vi "Parallel centroid calc (Optimized Performance) ajg.vi"() -> ()   [LabVIEW 2020]
doc: "The Parallel Processing (Optimized Performance) example shows how to process multiple images in parallel when using a ring acquisition. Images acquired from a camera are stored in a ring buffer and references to each image are pushed to a queue. Each worker loop removes a reference from the queue and processes the image.\n\nIn this example, image processing is simulated by a time delay that can be adjusted while the VI is running. When processing is complete, <B>IMAQdx Release Image</B> must be called in order to free space in the ring buffer."
uses:
  <vilib>/vision/driver/IMAQdx.llb/IMAQdx Acquisition Mode.ctl
  <vilib>/vision/Image Controls.llb/IMAQ Image.ctl
  <vilib>/vision/driver/IMAQdx.llb/IMAQdx Buffer Number Mode.ctl
  <vilib>/vision/driver/NI_Vision_Acquisition_Software.lvlib
  <resource>/objmgr/imaqdx.rc
panel:
  out "Images Saved Per Second":dbl
  out "Images Acquired Per Second":dbl
  out "Images Behind":u32
  in  "save path":path
  in  "Range":cluster{"Lower value":sgl, "Upper value":sgl}={"Lower value"=128.0, "Upper value"=255.0} {"Upper value" format="%.2f"; "Lower value" format="%.2f"}
  out "Lost Buffer Count":u32
  in  "Processing Delay (s)":dbl(slide)=0.1 scale=0.0..1.0
  out "Images Processed":u32
  out "Current Buffer Number":u32
  in  "Processing Delay (s)":dbl(slide)=0.2 scale=0.0..1.0
  out "Images Processed":u32
  out "Current Buffer Number":u32
  in  "Number of Images":i32=30
  out "Images in Queue":i32
  out "Images Processed":u32
  out "Current Buffer Number":u32
  in  "Camera Name":refnum<k21> caption="IMAQdx Session"
  in  "Stop":bool
  # "Overview: Demonstrates how to process multiple extracted images in parallel when using a ring acquisition.\nRequirements: Vision Acquisition Software\nInstructions:\n1. Select the Camera Name\n2. Run the VI"
  # "Worker Loop 1"
  # "Worker Loop 3"
  # "Worker Loop 2"
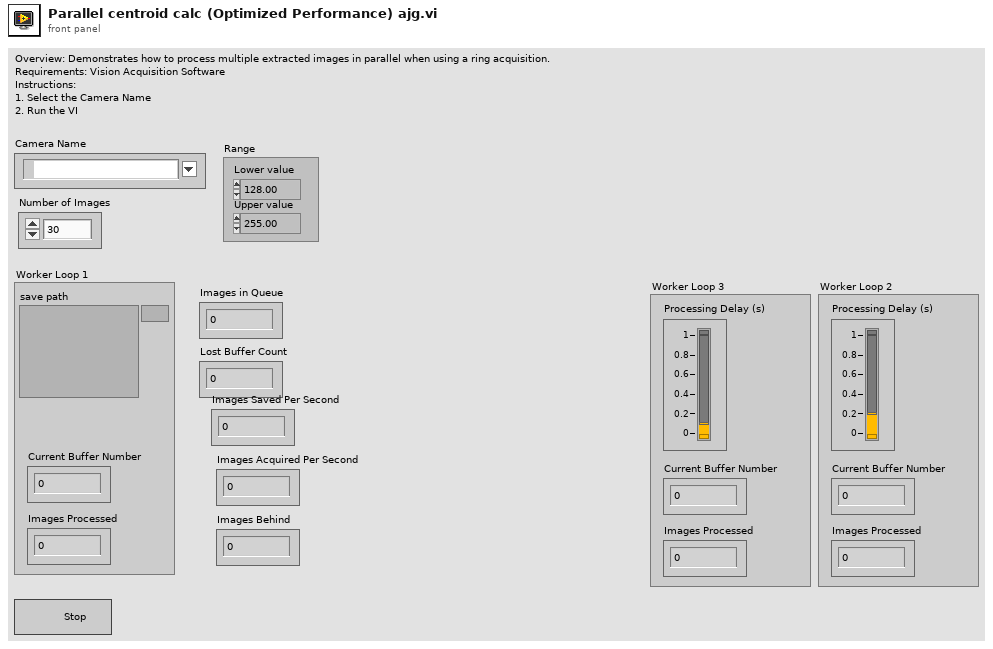
[diagram p1: front panel]
types:
  T1 = enum16{"open", "open or create", "create or replace", "create", "open (read-only)"}
  T2 = typedef "IMAQ Image.ctl" = refnum<image>
  T3 = typedef "NI_Vision_Acquisition_Software.lvlib/IMAQdx Acquisition Mode.ctl" = enum32{"One Shot", "Continuous"}
  T4 = typedef "IMAQdx.ctl" = refnum<k21>
  T5 = typedef "NI_Vision_Acquisition_Software.lvlib/IMAQdx Buffer Number Mode.ctl" = enum32{"Next", "Last", "Buffer Number", "Every", "Last New"}
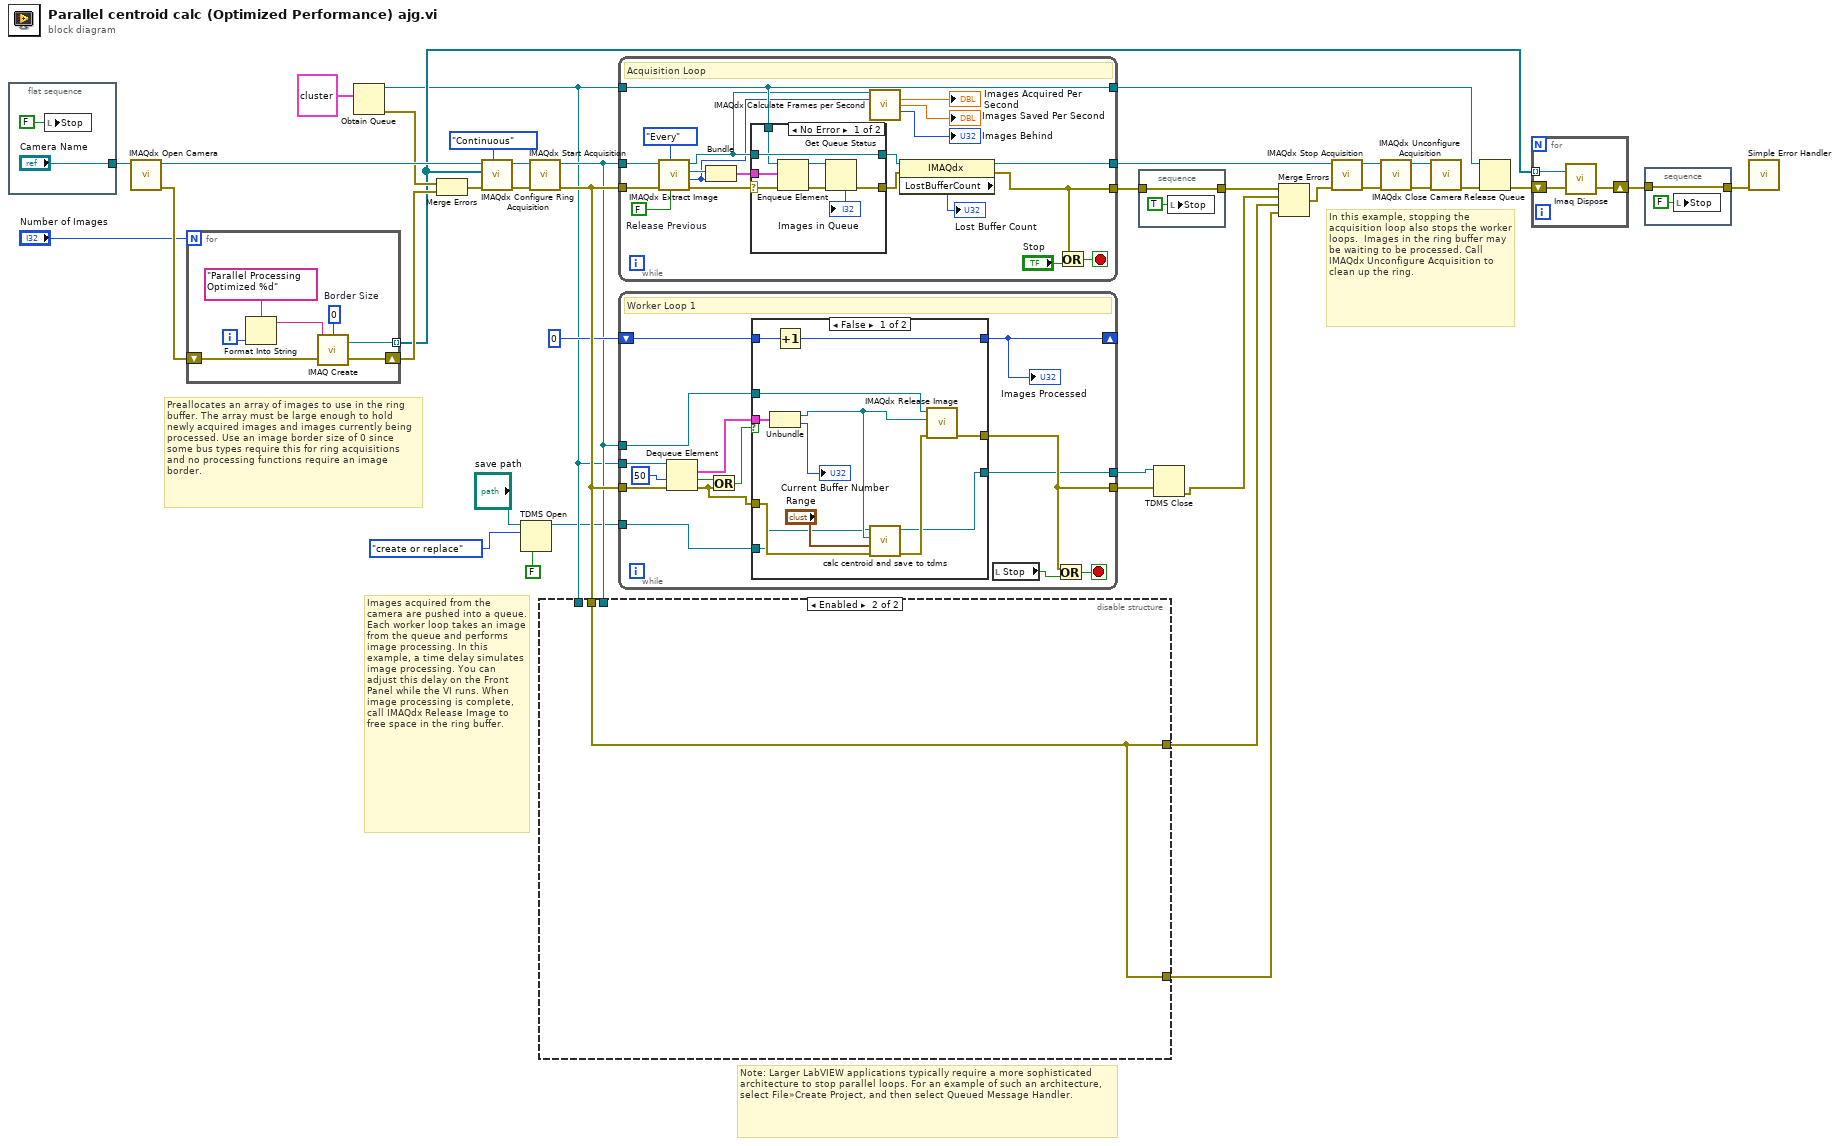
[diagram p0: block diagram]
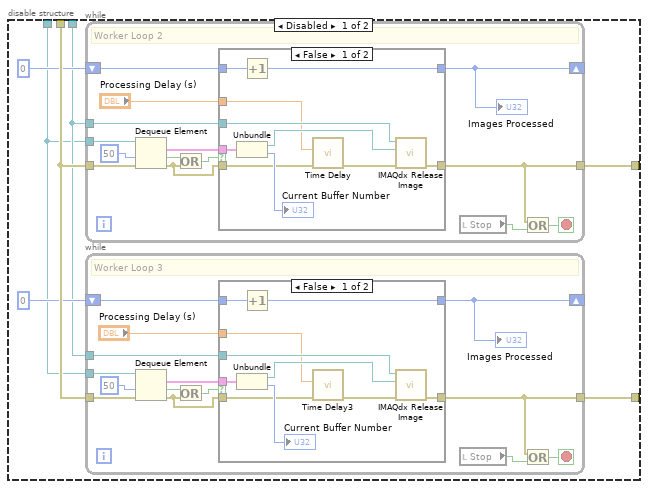
[diagram p2: hidden frame]
diagram:
  # "In this example, stopping the acquisition loop also stops the worker loops.  Images in the ring buffer may be waiting to be processed. Call IMAQdx Unconfigure Acquisition to clean up the ring."
  # "Images acquired from the camera are pushed into a queue. Each worker loop takes an image from the queue and performs image processing. In this example, a time delay simulates image processing. You can adjust this delay on the Front Panel while the VI runs. When image processing is complete, call IMAQdx Release Image to free space in the ring buffer."
  # "Preallocates an array of images to use in the ring buffer. The array must be large enough to hold newly acquired images and images currently being processed. Use an image border size of 0 since some bus types require this for ring acquisitions and no processing functions require an image border."
  # "Note: Larger LabVIEW applications typically require a more sophisticated architecture to stop parallel loops. For an example of such an architecture, select File»Create Project, and then select Queued Message Handler."
  n1 = flat-sequence {
    tunnel: ["Camera Name"] -> w36
    frame #0 {
      n2 = local write "Stop"(FALSE ("Stop")) -> ()
    }
  }
  n3 = call <vilib>:"IMAQdx Open Camera.vi"("Session In"=w36) -> ("error out"=w29:errorcluster, "Session Out"=w28:T4)  [unwired: 2 in, 7 out]
  n4 = for {
    N: "Number of Images" -> [_]
    tunnel: [w46] -> w19 mode=indexing
    shift-right: [w45] -> w24
    shift-left: w29 -> [w47]
    i -> [w44]
    w41 = 0  # Border Size
    n5 = Format Into String(format string="Parallel Processing Optimized %d" ("Image Name"), w44) -> (resulting string=w43:string)  [unwired: 2 in, 1 out]
    n6 = call "IMAQ Create"("Border Size"=w41, "Image Name"=w43, "error in (no error)"=w47) -> ("New Image"=w46:T2, "error out"=w45:errorcluster)  [unwired: 1 in, 1 out]
  }
  n7 = Obtain Queue(element data type=cluster{"Image Out":T2, "Buffer Number Out":u32} {"Image Out"=refnum, "Buffer Number Out"=0}) -> (queue out=w12:refnum<queue>, error out=w23:errorcluster)  [unwired: 4 in, 1 out]
  n8 = Merge Errors(w23, w24) -> (w25:errorcluster)
  n9 = call <vilib>:"IMAQdx Configure Ring Acquisition.vi"("Mode"=IMAQdx_Acquisition_Mode."Continuous" ("Continuous?"), "error in"=w25, "Images"=w19, "Session In"=w28) -> ("error out"=w30:errorcluster, "Session Out"=w31:T4)  [unwired: 5 in, 1 out]
  n10 = TDMS Open(6:FALSE ("disable buffering (T)"), 10:T1."create or replace" ("operation"), 11:"save path") -> (3:w4:refnum<k34>)  [unwired: 4 in, 1 out]
  n11 = call <vilib>:"IMAQdx Start Acquisition.vi"("error in"=w30, "Session In"=w31) -> ("error out"=w38:errorcluster, "Session Out"=w15:T4)  [unwired: 8 out]
  n12 = disable-structure shown="Enabled" {
    disable-tunnel: w38 -> [w54 w107]
    disable-tunnel: w15 -> [w51 _]
    disable-tunnel: [w50 w107] -> w14
    disable-tunnel: [w49 w107] -> w13
    disable-tunnel: w12 -> [w48 _]
    frame Disabled {
      n13 = while {
        tunnel: [w87] -> w50
        tunnel: w48 -> [w91]
        tunnel: w51 -> [w90]
        shift-right: [w85] -> _
        shift-left: u32 0 -> [w89]
        tunnel: w54 -> [w84]
        stop <- w93 stop-if-true
        # "Worker Loop 2"
        n14 = Dequeue Element(queue=w91, timeout in ms (-1)=50 ("timeout in ms"), error in (no error)=w84) -> (element=w92:cluster{"Image Out":T2, "Buffer Number Out":u32}, timed out?=w81:bool, error out=w82:errorcluster)  [unwired: 1 out]
        n15 = Or(x=w81, y=w82) -> (x .or. y?=w83:bool)
        n16 = case shown="False" w83 {
          tunnel: w92 -> [w104 _]
          tunnel: [w103 w105] -> w87
          tunnel: "Processing Delay (s)" -> [w97 _]
          tunnel: w90 -> [w100 _]
          tunnel: w89 -> [w99 w106]
          tunnel: [w98 w106] -> w85
          tunnel: w82 -> [w95 w105]
          frame False {
            n17 = Unbundle(w104) -> ("Image Out"=w101:T2, "Buffer Number Out"=→"Current Buffer Number":u32)
            n18 = Increment(x=w99) -> (x+1=w98:u32)
            n19 = call "Time Delay"("error in (no error)"=w95, "Delay Time (s)"=w97) -> ("error out"=w102:errorcluster)  [unwired: 9 in]
            n20 = call <vilib>:"IMAQdx Release Image.vi"("error in"=w102, "Image"=w101, "Session In"=w100) -> ("error out"=w103:errorcluster)  [unwired: 7 in, 1 out]
          }
          frame True {
            # "Empty queue or error.\nNothing to process."
          }
        }
        "Images Processed" <- w85
        n21 = local read "Stop"() -> (w88:bool)
        n22 = Or(x=w87, y=w88) -> (x .or. y?=w93:bool)
      }
      n23 = while {
        tunnel: [w61] -> w49
        tunnel: w48 -> [w65]
        tunnel: w51 -> [w64]
        shift-right: [w59] -> _
        shift-left: u32 0 -> [w63]
        tunnel: w54 -> [w58]
        stop <- w67 stop-if-true
        # "Worker Loop 3"
        n24 = Dequeue Element(queue=w65, timeout in ms (-1)=50 ("timeout in ms"), error in (no error)=w58) -> (element=w66:cluster{"Image Out":T2, "Buffer Number Out":u32}, timed out?=w57:bool, error out=w55:errorcluster)  [unwired: 1 out]
        n25 = Or(x=w57, y=w55) -> (x .or. y?=w56:bool)
        n26 = case shown="False" w56 {
          tunnel: w66 -> [w78 _]
          tunnel: [w77 w79] -> w61
          tunnel: "Processing Delay (s)" -> [w71 _]
          tunnel: w64 -> [w74 _]
          tunnel: w63 -> [w73 w80]
          tunnel: [w72 w80] -> w59
          tunnel: w55 -> [w69 w79]
          frame False {
            n27 = Unbundle(w78) -> ("Image Out"=w75:T2, "Buffer Number Out"=→"Current Buffer Number":u32)
            n28 = Increment(x=w73) -> (x+1=w72:u32)
            n29 = call "Time Delay3"("error in (no error)"=w69, "Delay Time (s)"=w71) -> ("error out"=w76:errorcluster)  [unwired: 9 in]
            n30 = call <vilib>:"IMAQdx Release Image.vi"("error in"=w76, "Image"=w75, "Session In"=w74) -> ("error out"=w77:errorcluster)  [unwired: 7 in, 1 out]
          }
          frame True {
            # "Empty queue or error.\nNothing to process."
          }
        }
        "Images Processed" <- w59
        n31 = local read "Stop"() -> (w62:bool)
        n32 = Or(x=w61, y=w62) -> (x .or. y?=w67:bool)
      }
    }
    frame Enabled {
    }
  }
  n33 = while {
    tunnel: w38 -> [w127]
    tunnel: w15 -> [w123]
    tunnel: w12 -> [w114]
    tunnel: [w122] -> w18
    tunnel: [w120] -> w11
    tunnel: [w114] -> w20
    stop <- w119 stop-if-true
    w124 = FALSE  # Release Previous
    # "Acquisition Loop"
    n34 = call <vilib>:"IMAQdx Extract Image.vi"("Release Previous (true)"=w124, "Buffer Number Mode (Next)"=IMAQdx_Buffer_Number_Mode."Every" ("Buffer Number Mode"), "error in"=w127, "Session In"=w123) -> ("error out"=w118:errorcluster, "Buffer Number Out"=w108:u32, "Image Out"=w117:T2, "Session Out"=w109:T4)  [unwired: 4 in]
    n35 = Bundle("Image Out"=w117, "Buffer Number Out"=w108) -> (w115:cluster{"Image Out":T2, "Buffer Number Out":u32})  [unwired: 1 in]
    n36 = case shown="No Error" w118 {
      selector: w118 -> [w131 w136]
      tunnel: [w132 w137] -> w116
      tunnel: w109 -> [w132 w137]
      tunnel: w115 -> [w130 _]
      tunnel: w114 -> [w129 _]
      tunnel: [w128 w136] -> w113
      frame No Error {
        n37 = Enqueue Element(queue=w129, element=w130, error in (no error)=w131) -> (queue out=w134:refnum<queue>, error out=w135:errorcluster)  [unwired: 1 in, 1 out]
        n38 = Get Queue Status(queue=w134, error in (no error)=w135) -> (error out=w128:errorcluster, # elements in queue=→"Images in Queue":i32)  [unwired: 1 in, 6 out]
      }
      frame Error {
      }
    }
    n39 = call <vilib>:"IMAQdx Calculate Frames per Second.vi"("Session In"=w109, "Buffer Number"=w108) -> ("Acquired Frames per Second"=→"Images Acquired Per Second":dbl, "Processed Frames per Second"=→"Images Saved Per Second":dbl, "Images Behind"=→"Images Behind":i32)  [unwired: 7 in, 4 out]
    n40 = property class="IMAQdx"(reference=w116, error in=w113) -> (reference out=w122:T4, error out=w120:errorcluster, "LostBufferCount"=→"Lost Buffer Count":u32)
    n41 = Or(x=w120, y="Stop") -> (x .or. y?=w119:bool)
  }
  n42 = while {
    tunnel: [w145] -> w2
    tunnel: w12 -> [w149]
    tunnel: w15 -> [w148]
    shift-right: [w144] -> _
    shift-left: u32 0 -> [w147]
    tunnel: w38 -> [w143]
    tunnel: w4 -> [w139]
    tunnel: [w138] -> w3
    stop <- w151 stop-if-true
    # "Worker Loop 1"
    n43 = Dequeue Element(queue=w149, timeout in ms (-1)=50 ("timeout in ms"), error in (no error)=w143) -> (element=w150:cluster{"Image Out":T2, "Buffer Number Out":u32}, timed out?=w141:bool, error out=w140:errorcluster)  [unwired: 1 out]
    n44 = Or(x=w141, y=w140) -> (x .or. y?=w142:bool)
    n45 = case shown="False" w142 {
      tunnel: w140 -> [w156 w167]
      tunnel: w150 -> [w164 _]
      tunnel: [w163 w167] -> w145
      tunnel: w148 -> [w162 _]
      tunnel: w147 -> [w160 w166]
      tunnel: [w159 w166] -> w144
      tunnel: w139 -> [w154 w165]
      tunnel: [w153 w165] -> w138
      frame False {
        n46 = Unbundle(w164) -> ("Image Out"=w158:T2, "Buffer Number Out"=→"Current Buffer Number":u32)
        n47 = Increment(x=w160) -> (x+1=w159:u32)
        n48 = call "calc centroid and save to tdms.vi"("error in (no error)"=w156, "Range"="Range", "Image Out"=w158, "Refnum in"=w154) -> ("error out"=w155:errorcluster, "Refnum out"=w153:refnum<k34>)  [unwired: 6 in]
        n49 = call <vilib>:"IMAQdx Release Image.vi"("error in"=w155, "Image"=w158, "Session In"=w162) -> ("error out"=w163:errorcluster)  [unwired: 7 in, 1 out]
      }
      frame True {
        # "Empty queue or error.\nNothing to process."
      }
    }
    "Images Processed" <- w144
    n50 = local read "Stop"() -> (w146:bool)
    n51 = Or(x=w145, y=w146) -> (x .or. y?=w151:bool)
  }
  n52 = stacked-sequence {
    tunnel: [w168] -> w10
    tunnel: w11 -> [w168]
    frame #0 {
      n53 = local write "Stop"(TRUE ("Stop")) -> ()
    }
  }
  n54 = TDMS Close(8:w2, 11:w3) -> (0:w1:errorcluster)  [unwired: 1 out]
  n55 = Merge Errors(w10, w1, w14, w13) -> (w22:errorcluster)
  n56 = call <vilib>:"IMAQdx Stop Acquisition.vi"("error in"=w22, "Session In"=w18) -> ("error out"=w32:errorcluster, "Session Out"=w33:T4)  [unwired: 8 out]
  n57 = call <vilib>:"IMAQdx Unconfigure Acquisition.vi"("error in"=w32, "Session In"=w33) -> ("error out"=w35:errorcluster, "Session Out"=w34:T4)  [unwired: 8 out]
  n58 = call <vilib>:"IMAQdx Close Camera.vi"("error in"=w35, "Session In"=w34) -> ("error out"=w17:errorcluster)  [unwired: 9 out]
  n59 = Release Queue(queue=w20, error in (no error)=w17) -> (error out=w16:errorcluster)  [unwired: 1 in, 2 out]
  n60 = for {
    shift-right: [w171] -> w9
    shift-left: w16 -> [w172]
    tunnel: w19 -> [w170] mode=indexing
    n61 = call "Imaq Dispose"("Image"=w170, "error in (no error)"=w172) -> ("error out"=w171:errorcluster)  [unwired: 4 in]
  }
  n62 = stacked-sequence {
    tunnel: [w173] -> w8
    tunnel: w9 -> [w173]
    frame #0 {
      n63 = local write "Stop"(FALSE ("Stop")) -> ()
    }
  }
  n64 = call <vilib>:"Simple Error Handler.vi"("error in (no error)"=w8) -> ()  [unwired: 4 in, 5 out]
